vi "E70 Sunshade Color Configuration.vi"(11 "Base Path":path) -> ()   [LabVIEW 2018]
uses:
  02.Type Def's/Sunshade Color Configuration Cluster.ctl
panel:
  in  "Save":bool
  in  "Exit":bool
  in  "Array":T1[](array[typedef])
  # "Sunshade Color Configuration"
  # "Keyence Tuning\nParameter Bank Index"
  # "PLC Sunshade 1"
  # "PLC Sunshade 2"
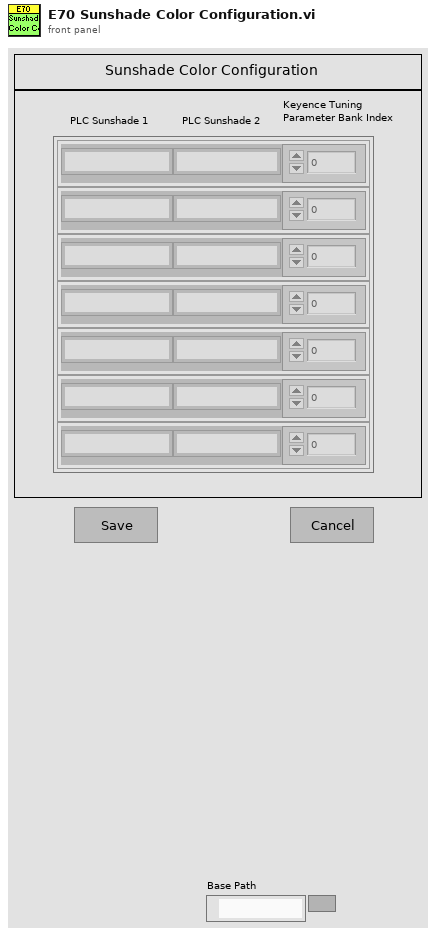
[diagram p1: front panel]
types:
  T1 = typedef "Sunshade Color Configuration Cluster.ctl" = cluster{"Sunshade 1 Number":string, "Sunshade 2 Number":string, "keyence tuning bank param idx":i32}
  T2 = cluster{"Array":T1[], "Base Path":path, "File Path":path}
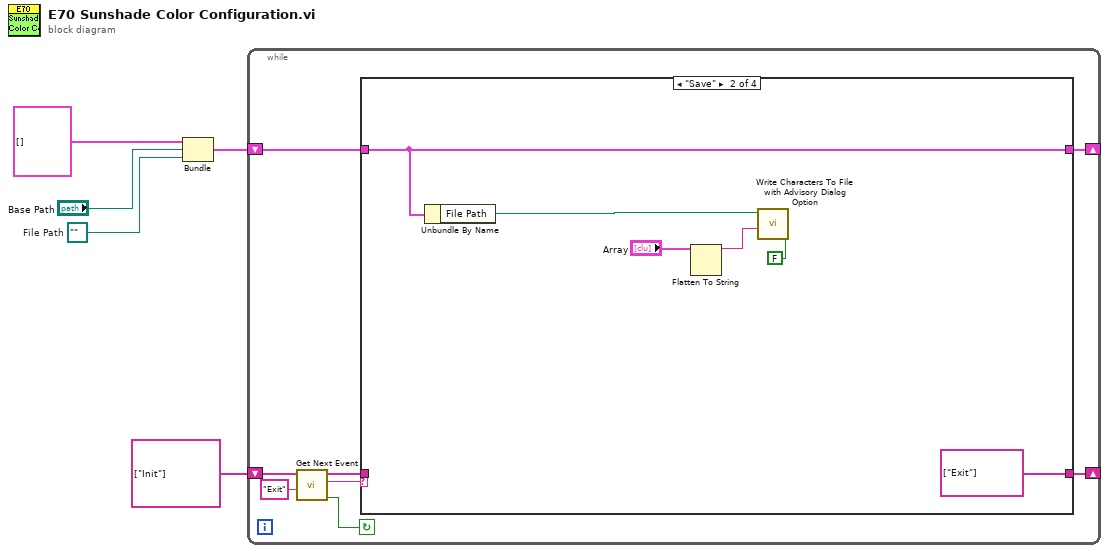
[diagram p0: block diagram]
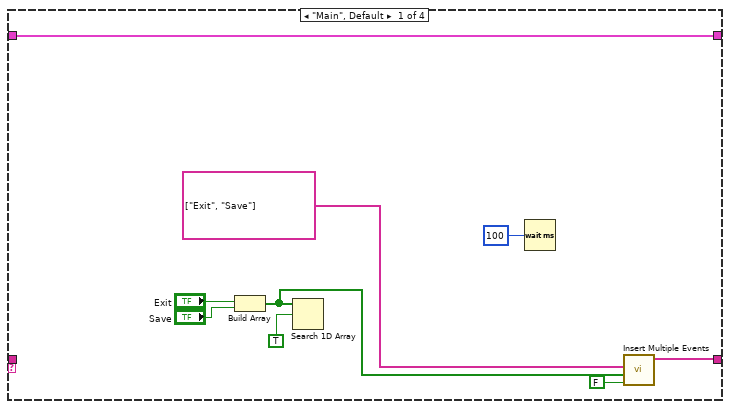
[diagram p2: hidden frame]
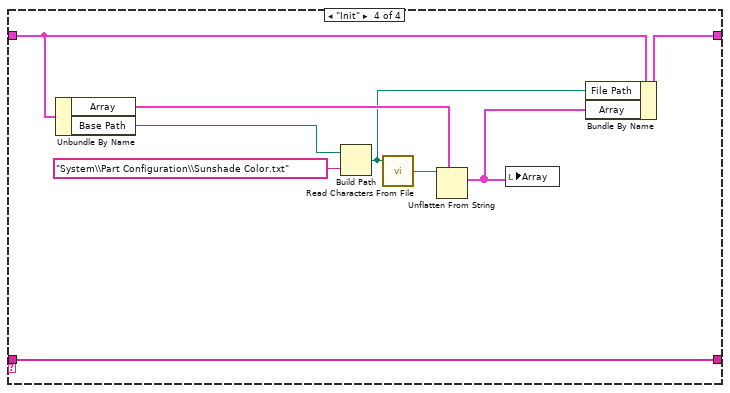
[diagram p4: hidden frame]
diagram:
  w1 = path ""  # File Path
  n1 = Bundle("Array"=T1[] [], "Base Path"="Base Path", "File Path"=w1) -> (w4:T2)  [unwired: 1 in]
  n2 = while {
    shift-right: [w11] -> _
    shift-left: string[] ["Init"] ("Event queue out") -> [w10]
    shift-right: [w6] -> _
    shift-left: w4 -> [w7]
    stop <- w9 continue-if-true
    n3 = call "Get Next Event.vi"("Exit Event"="Exit", "event queue in"=w10) -> ("Condition (Exit:F)"=w9:bool, "next event"=w13:string, "event queue out"=w12:string[])  [unwired: 3 in]
    n4 = case shown="\"Save\"" w13 {
      tunnel: w12 -> [_ _ w30 w39]
      tunnel: [w21 string[] ["Exit"] ("Event queue out") w30 w39] -> w11
      tunnel: w7 -> [w16 w27 w29 w36]
      tunnel: [w16 w27 w29 w38] -> w6
      frame "Main", Default {
        n5 = Build Array("Exit", "Save") -> (w19:bool[])
        n6 = Search 1D Array(1D array=w19, element=TRUE) -> ()  [unwired: 1 in, 1 out]
        n7 = Wait (ms)(milliseconds to wait=u32 100) -> ()  [unwired: 1 out]
        n8 = call "Insert Multiple Events.vi"("Insert all? (T)"=FALSE, "Insert Selected?"=w19, "Events to Insert"=string[] ["Exit", "Save"]) -> ("Event queue out"=w21:string[])  [unwired: 4 in]
      }
      frame "Save" {
        n9 = Unbundle By Name(w27) -> ("File Path"=w25:path)
        n10 = Flatten To String(anything="Array") -> (data string=w24:string)  [unwired: 3 in, 2 out]
        n11 = call "Write Characters To File with Advisory Dialog Option.vi"("advisory dialog? (display:T)"=FALSE, "character string"=w24, "file path (dialog if empty)"=w25) -> ()  [unwired: 7 in, 2 out]
      }
      frame "Exit" {
      }
      frame "Init" {
        n12 = Unbundle By Name(w36) -> ("Array"=w34:T1[], "Base Path"=w35:path)
        n13 = Build Path(base path=w35, name or relative path="System\\Part Configuration\\Sunshade Color.txt") -> (appended path=w32:path)
        n14 = call <vilib>:"Read Characters From File.vi"("file path (dialog if empty)"=w32) -> ("character string"=w37:string)  [unwired: 5 in, 3 out]
        n15 = Unflatten From String(type=w34, binary string=w37) -> (value=w31:T1[])  [unwired: 3 in, 2 out]
        n16 = local write "Array"(w31) -> ()
        n17 = Bundle By Name(cluster=w36, "File Path"=w32, "Array"=w31) -> (w38:T2)
      }
    }
  }
